vi "RSZVB Get RGB Color.vi"(8 "error in (no error)":errorcluster {"code" format="%.0x"}, 10 "Element (1: Background)":i32(ring)=1 items=["Background"=1, "Text"=2, "Selected Text"=3, "Grid"=4, "Reference Line"=5, "Same Color for all Markers"=0, "Horizontal Line / Vertical Range Lines"=7, "Diagram Title"=8, "Limit Fail Trace Color"=9, "Limit Line Type Off"=10, "Limit Line Type Upper"=11, "Limit Line Type Lower"=12, "Trace 1"=13, "Trace 2"=14, "Trace 3"=15, "Trace 4"=16, "Trace 5"=17, "Trace 6"=18, "Trace 7"=19, "Trace 8"=20, "Trace 9"=21, "Trace 10"=22, "Trace 11"=23, "Trace 12"=24, "Trace 13"=25, "Trace 14"=26, "Trace 15"=27, "Trace 16"=28], 11 "VISA session":refnum<visa-resource-name>) -> (0 "error out":errorcluster {"code" format="%.0x"}, 1 "Red":dbl format="%^.3e", 3 "dup VISA session":refnum<visa-resource-name>, 4 "Trace Style (0: Solid)":i32, 5 "Blue":dbl format="%^.3e", 6 "Green":dbl format="%^.3e", 7 "Trace Width (1)":i32)   [LabVIEW 2011]
doc: "This VI returns color of all display elements based on the Red/Green/Blue color model. \n\nRemote-control command(s):\nDISPlay:CMAP<Element>:RGB?"
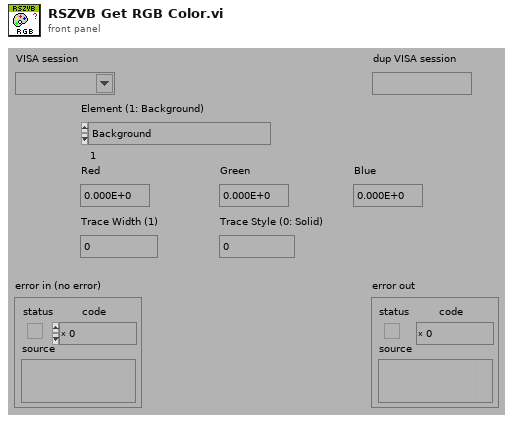
[diagram p1: front panel]
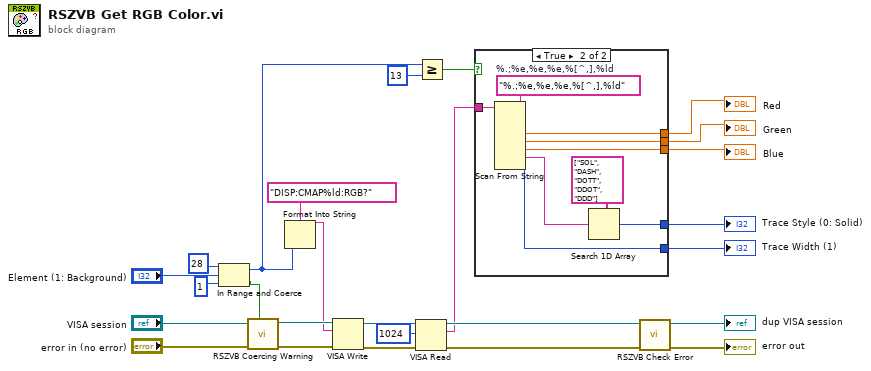
[diagram p0: block diagram]
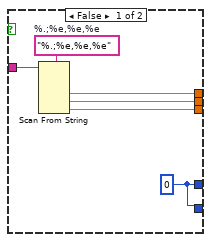
[diagram p2: hidden frame]
diagram:
  n1 = In Range and Coerce(upper limit=28 ("lower limit"), x="Element (1: Background)", lower limit=1) -> (coerced(x)=w8:i32, In Range?=w12:bool)
  n2 = call "RSZVB Coercing Warning.vi"("In Range?"=w12, "error in (no error)"="error in (no error)", "VISA session"="VISA session") -> ("error out"=w24:errorcluster, "dup VISA session"=w25:refnum<visa-resource-name>)  [unwired: 7 in]
  n3 = Format Into String(format string="DISP:CMAP%ld:RGB?", w8) -> (resulting string=w23:string)  [unwired: 2 in, 1 out]
  n4 = VISA Write(VISA resource name=w25, write buffer=w23, error in (no error)=w24) -> (VISA resource name out=w17:refnum<visa-resource-name>, error out=w18:errorcluster)  [unwired: 1 out]
  n5 = VISA Read(VISA resource name=w17, byte count=u32 1024 ("byte count (0)"), error in (no error)=w18) -> (VISA resource name out=w21:refnum<visa-resource-name>, read buffer=w1:string, error out=w20:errorcluster)  [unwired: 1 out]
  n6 = Greater Or Equal?(x=w8, y=13) -> (x >= y?=w4:bool)
  n7 = case shown="True" w4 {
    tunnel: w1 -> [w27 w40]
    tunnel: [w31 w39] -> w7
    tunnel: [w30 w38] -> w6
    tunnel: [w29 w37] -> w5
    tunnel: [w28 w35] -> w3
    tunnel: [w28 w34] -> w2
    frame False {
      w28 = 0
      w32 = "%.;%e,%e,%e"  # %.;%e,%e,%e
      n8 = Scan From String(format string=w32, input string=w27) -> (output 1=w31:dbl, output 2=w30:dbl, output 3=w29:dbl)  [unwired: 5 in, 3 out]
    }
    frame True {
      w41 = "%.;%e,%e,%e,%[^,],%ld"  # %.;%e,%e,%e,%[^,],%ld
      n9 = Scan From String(format string=w41, input string=w40) -> (output 1=w39:dbl, output 2=w38:dbl, output 3=w37:dbl, output 4=w33:string, output 5=w34:i32)  [unwired: 7 in, 3 out]
      n10 = Search 1D Array(1D array=string[] ["SOL", "DASH", "DOTT", "DDOT", "DDD"] ("array 2"), element=w33) -> (index of element=w35:i32)  [unwired: 1 in]
    }
  }
  "Red" <- w7
  "Green" <- w6
  "Blue" <- w5
  "Trace Style (0: Solid)" <- w3
  "Trace Width (1)" <- w2
  n11 = call "RSZVB Check Error.vi"("error in (no error)"=w20, "VISA session"=w21) -> ("error out"=→"error out":errorcluster, "dup VISA session"=→"dup VISA session":refnum<visa-resource-name>)  [unwired: 8 in]
